vi "Initialize and Clear Graph.vi"(8 "error in (no error)":errorcluster, 9 "Record Name Prefix":string, 10 "Max Visible Legend":i32=-1, 11 "WaveformGraph Ref":refnum<vi>) -> (0 "error out":errorcluster, 3 "Live Graph Plotter out":refnum<class "Live Graph Plotter.lvclass">)   [LabVIEW 2025, in "Live Graph Plotter.lvclass"]
uses:
  Live Graph Plotter.lvclass
  Live Graph Plotter.lvclass/Live Graph Plotter.ctl
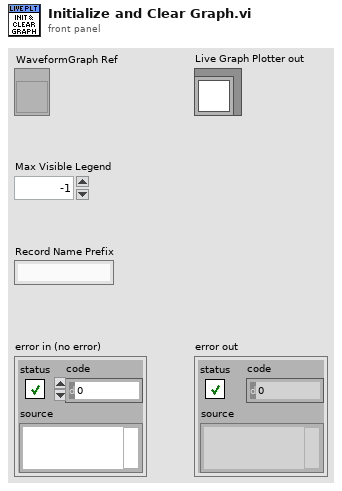
[diagram p1: front panel]
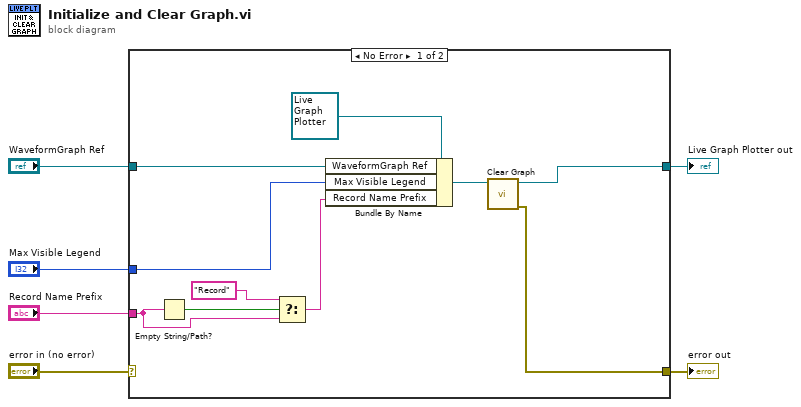
[diagram p0: block diagram]
diagram:
  n1 = case shown="No Error" "error in (no error)" {
    selector: "error in (no error)" -> [_ w17]
    tunnel: [w7 w17] -> w5
    tunnel: "WaveformGraph Ref" -> [w14 _]
    tunnel: [w8 _] -> w3
    tunnel: "Max Visible Legend" -> [w13 _]
    tunnel: "Record Name Prefix" -> [w11 _]
    frame No Error {
      n2 = Empty String/Path?(string/path=w11) -> (empty?=w10:bool)
      n3 = Select(t="Record", s=w10, f=w11) -> (s? t:f=w12:string)
      n4 = Bundle By Name(cluster=refnum<class "Live Graph Plotter.lvclass"> refnum ("Live Graph Plotter.lvclass"), "WaveformGraph Ref"=w14, "Max Visible Legend"=w13, "Record Name Prefix"=w12) -> (w15:refnum<class "Live Graph Plotter.lvclass">)
      n5 = call "Clear Graph.vi"("Live Graph Plotter in"=w15) -> ("error out"=w7:errorcluster, "Live Graph Plotter out"=w8:refnum<class "Live Graph Plotter.lvclass">)  [unwired: 9 in]
    }
    frame Error {
    }
  }
  "error out" <- w5
  "Live Graph Plotter out" <- w3
